vi "example_01_download.vi"() -> ()   [LabVIEW 2015, in "lv-bin-wget.lvlib" / "v1.lvlib"]
uses:
  v1.lvlib
  <userlib>/antonio-alexander/lv-bin/lv-bin/public/api/v1/advanced/add_data_path_multiple.vi
  <userlib>/antonio-alexander/lv-bin/lv-bin/public/api/v1/v1.lvlib
panel:
  out "error out":errorcluster
  in  "address":string
  in  "target_path":path
  in  "bin_path":path
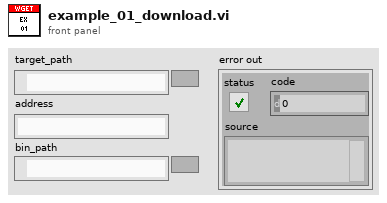
[diagram p1: front panel]
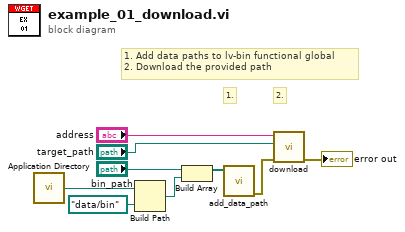
[diagram p0: block diagram]
diagram:
  # "1. Add data paths to lv-bin functional global\n2. Download the provided path"
  # "2."
  # "1."
  n1 = call <vilib>:"Application Directory.vi"() -> ("Application Directory"=w6:path)
  n2 = Build Path(base path=w6, name or relative path=path "data/bin" ("Application Directory")) -> (appended path=w7:path)
  n3 = Build Array("bin_path", w7) -> (w8:path[])
  n4 = call-poly <userlib>:"add_data_path.vi"("path_to_add []"=w8) -> ("error out"=w4:errorcluster)  [unwired: 10 in]
  n5 = call "download.vi"("error in (no error)"=w4, "target_path"="target_path", "address"="address") -> ("error out"=→"error out":errorcluster)  [unwired: 8 in]
